vi "run_Ix.vi"() -> ()   [LabVIEW 2020]
panel:
  out "a+b":dbl[](array[numeric])
  in  "protocol_type":dbl
  in  "end_time":dbl
  in  "ip_recv":string
  in  "ip_send":string
  in  "runpath":string
  out "error out":errorcluster caption="错误输出"
  in  "recv_count":dbl
  in  "send_count":dbl
  in  "路径":path
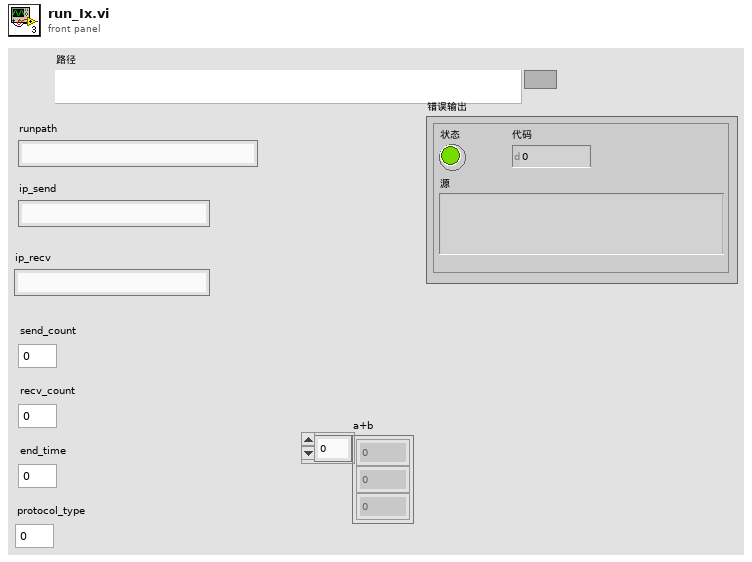
[diagram p1: front panel]
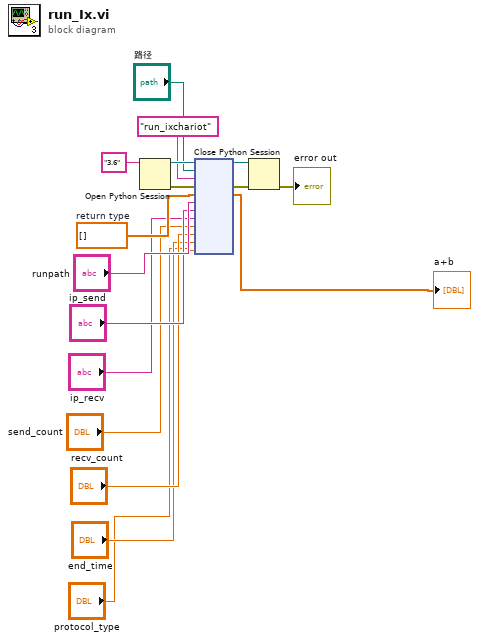
[diagram p0: block diagram]
diagram:
  w8 = dbl[] []  # return type
  n1 = Open Python Session(python version="3.6") -> (session out=w16:refnum<k35>, error out=w12:errorcluster)  [unwired: 2 in]
  n2 = node(w16, "路径", "run_ixchariot", w12, w8, "runpath", "ip_send", "ip_recv", "send_count", "recv_count", "end_time", "protocol_type") -> (w15:refnum<k35>, w11:errorcluster, →"a+b":dbl[])  [unwired: 7 in, 2 out]
  n3 = Close Python Session(session in=w15, error in=w11) -> (11:→"error out":errorcluster)
